vi "Read_Master_Config.vi"(4 "error in (no error)":errorcluster, 7 "configuration file path":path) -> (0 "error out":errorcluster, 1 "Valid INI?":bool, 2 "Present Configuration":T1)   [LabVIEW 2015]
uses:
  <vilib>/Utility/config.llb/Read Key (String).vi
  <vilib>/Utility/config.llb/NI_LVConfig.lvlib
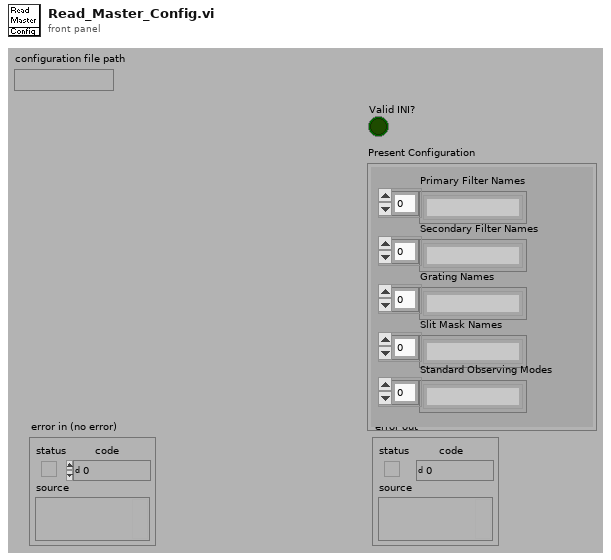
[diagram p1: front panel]
types:
  T1 = cluster{"Primary Filter Names":string[], "Secondary Filter Names":string[], "Grating Names":string[], "Slit Mask Names":string[], "Standard Observing Modes":string[]}
  T2 = typedef "NI_LVConfig.lvlib/Config Data RefNum.ctl" = refnum<k1>
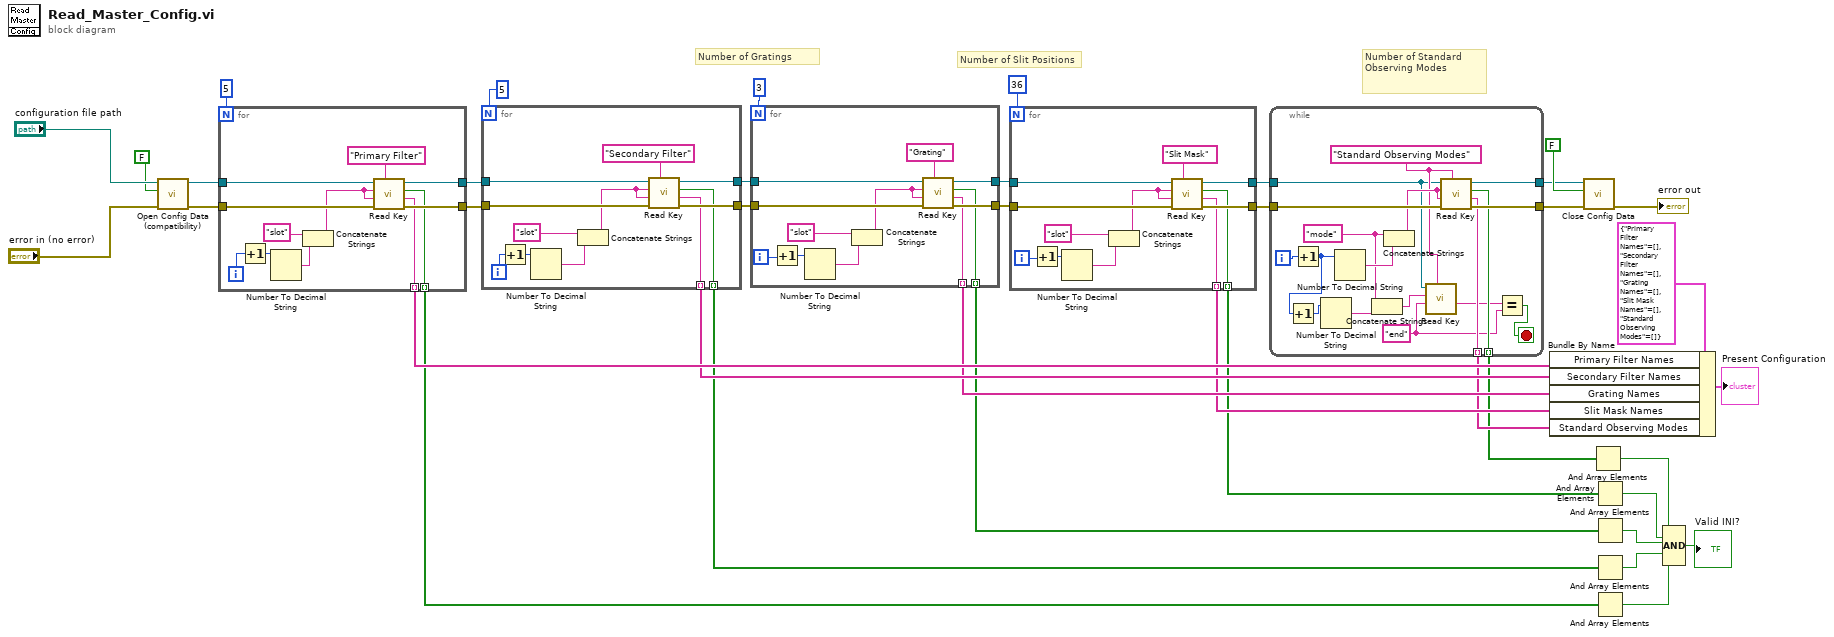
[diagram p0: block diagram]
diagram:
  # "Number of Gratings"
  # "Number of Slit Positions"
  # "Number of Standard Observing Modes"
  n1 = call <vilib>:"Open Config Data (compatibility).vi"("error in (no error)"="error in (no error)", "create file if necessary (T)"=FALSE, "configuration file path"="configuration file path") -> ("error out"=w36:errorcluster, "refnum"=w35:T2)  [unwired: 6 in, 1 out]
  n2 = for {
    N: 5 -> [_]
    tunnel: w36 -> [w51]
    tunnel: w35 -> [w50]
    tunnel: [w46] -> w34
    tunnel: [w45] -> w33
    tunnel: [w43] -> w22 mode=indexing
    tunnel: [w42] -> w26 mode=indexing
    i -> [w41]
    n3 = Increment(x=w41) -> (x+1=w40:i32)
    n4 = Number To Decimal String(number=w40) -> (decimal integer string=w48:string)  [unwired: 1 in]
    n5 = Concatenate Strings("slot", w48) -> (w44:string)
    n6 = call-poly <vilib>:"Read Key.vi"("section"="Primary Filter", "error in (no error)"=w51, "default value"=w44, "key"=w44, "refnum"=w50) -> ("error out"=w46:errorcluster, "value"=w42:string, "found?"=w43:bool, "refnum out"=w45:T2)  [unwired: 3 in]
  }
  n7 = for {
    N: 5 -> [_]
    tunnel: w34 -> [w63]
    tunnel: w33 -> [w62]
    tunnel: [w58] -> w32
    tunnel: [w57] -> w31
    tunnel: [w55] -> w21 mode=indexing
    tunnel: [w54] -> w25 mode=indexing
    i -> [w53]
    n8 = Increment(x=w53) -> (x+1=w52:i32)
    n9 = Number To Decimal String(number=w52) -> (decimal integer string=w60:string)  [unwired: 1 in]
    n10 = Concatenate Strings("slot", w60) -> (w56:string)
    n11 = call-poly <vilib>:"Read Key.vi"("section"="Secondary Filter", "error in (no error)"=w63, "default value"=w56, "key"=w56, "refnum"=w62) -> ("error out"=w58:errorcluster, "value"=w54:string, "found?"=w55:bool, "refnum out"=w57:T2)  [unwired: 3 in]
  }
  n12 = for {
    N: 3 -> [_]
    tunnel: w32 -> [w75]
    tunnel: w31 -> [w74]
    tunnel: [w70] -> w29
    tunnel: [w69] -> w30
    tunnel: [w67] -> w20 mode=indexing
    tunnel: [w66] -> w24 mode=indexing
    i -> [w64]
    n13 = Increment(x=w64) -> (x+1=w65:i32)
    n14 = Number To Decimal String(number=w65) -> (decimal integer string=w72:string)  [unwired: 1 in]
    n15 = Concatenate Strings("slot", w72) -> (w68:string)
    n16 = call-poly <vilib>:"Read Key.vi"("section"="Grating", "error in (no error)"=w75, "default value"=w68, "key"=w68, "refnum"=w74) -> ("error out"=w70:errorcluster, "value"=w66:string, "found?"=w67:bool, "refnum out"=w69:T2)  [unwired: 3 in]
  }
  n17 = for {
    N: 36 -> [_]
    tunnel: w29 -> [w87]
    tunnel: w30 -> [w86]
    tunnel: [w82] -> w8
    tunnel: [w81] -> w9
    tunnel: [w79] -> w19 mode=indexing
    tunnel: [w78] -> w23 mode=indexing
    i -> [w77]
    n18 = Increment(x=w77) -> (x+1=w76:i32)
    n19 = Number To Decimal String(number=w76) -> (decimal integer string=w84:string)  [unwired: 1 in]
    n20 = Concatenate Strings("slot", w84) -> (w80:string)
    n21 = call-poly <vilib>:"Read Key.vi"("section"="Slit Mask", "error in (no error)"=w87, "default value"=w80, "key"=w80, "refnum"=w86) -> ("error out"=w82:errorcluster, "value"=w78:string, "found?"=w79:bool, "refnum out"=w81:T2)  [unwired: 3 in]
  }
  n22 = while {
    tunnel: w8 -> [w105]
    tunnel: w9 -> [w88]
    tunnel: [w103] -> w6
    tunnel: [w102] -> w7
    tunnel: [w101] -> w3 mode=indexing
    tunnel: [w100] -> w5 mode=indexing
    i -> [w97]
    stop <- w99 stop-if-true
    w91 = "end"
    w93 = "mode"
    w89 = "Standard Observing Modes" ("section")
    n23 = Increment(x=w97) -> (x+1=w96:i32)
    n24 = Increment(x=w96) -> (x+1=w95:i32)
    n25 = Number To Decimal String(number=w95) -> (decimal integer string=w94:string)  [unwired: 1 in]
    n26 = Number To Decimal String(number=w96) -> (decimal integer string=w104:string)  [unwired: 1 in]
    n27 = Concatenate Strings(w93, w94) -> (w92:string)
    n28 = Concatenate Strings(w93, w104) -> (w98:string)
    n29 = call-poly <vilib>:"Read Key.vi"("section"=w89, "default value"=w91, "key"=w92, "refnum"=w88) -> ("value"=w90:string)  [unwired: 4 in, 3 out]
    n30 = call-poly <vilib>:"Read Key.vi"("section"=w89, "error in (no error)"=w105, "default value"=w98, "key"=w98, "refnum"=w88) -> ("error out"=w103:errorcluster, "value"=w100:string, "found?"=w101:bool, "refnum out"=w102:T2)  [unwired: 3 in]
    n31 = Equal?(x=w90, y=w91) -> (x = y?=w99:bool)
  }
  n32 = Bundle By Name(cluster=T1 {"Primary Filter Names"=[], "Secondary Filter Names"=[], "Grating Names"=[], "Slit Mask Names"=[], "Standard Observing Modes"=[]} ("Present Configuration"), "Primary Filter Names"=w26, "Secondary Filter Names"=w25, "Grating Names"=w24, "Slit Mask Names"=w23, "Standard Observing Modes"=w5) -> (→"Present Configuration":T1)
  n33 = call <vilib>:"Close Config Data.vi"("error in (no error)"=w6, "write file if changed (T)"=FALSE, "refnum"=w7) -> ("error out"=→"error out":errorcluster)  [unwired: 7 in, 1 out]
  n34 = And Array Elements(Boolean array=w3) -> (logical AND=w4:bool)
  n35 = And Array Elements(Boolean array=w19) -> (logical AND=w18:bool)
  n36 = And Array Elements(Boolean array=w20) -> (logical AND=w15:bool)
  n37 = And Array Elements(Boolean array=w21) -> (logical AND=w16:bool)
  n38 = And Array Elements(Boolean array=w22) -> (logical AND=w17:bool)
  n39 = Compound Arithmetic op=AND(w4, w18, w15, w16, w17) -> (→"Valid INI?":bool)
